vi "Helmholtz2D_FEM_Check Input_RHS.vi"(8 "error in (no error)":errorcluster, 10 "Grid":cluster{"Xi":dbl[], "Yi":dbl[]}, 11 "F(x, y)":dbl[](array[numeric])) -> (0 "error out":errorcluster)   [LabVIEW 2017, in "NI_PDE.lvlib"]
uses:
  <vilib>/gmath/NI_PDE.lvlib
  <vilib>/gmath/pde.llb/Common/PDE_Error.ctl
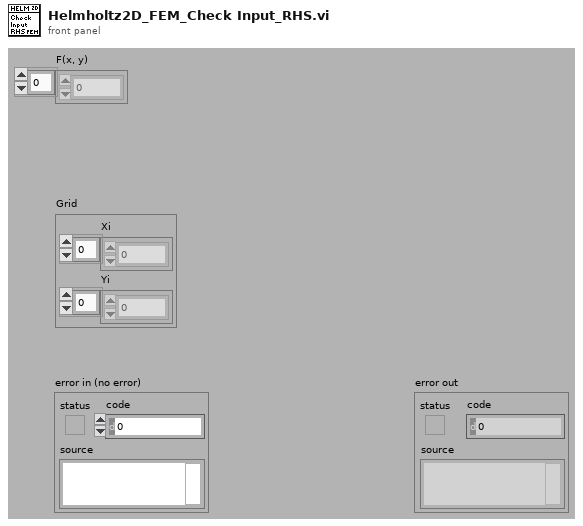
[diagram p1: front panel]
types:
  T1 = typedef "NI_PDE.lvlib/PDE_Error.ctl" = enum16{"No Error", "k is zero", "End point <= start point", "# of time steps < 2", "# of spatial points < 3", "# of grid < 1 for FEM", "# of boundary < 3 for FEM", "Incompatible RHS size", "Incompatible BC size", "Incompatible IC size", "PDE class conflict", "RHS class conflict", "Domain class conflict", "BC class conflict", "IC class conflict"}
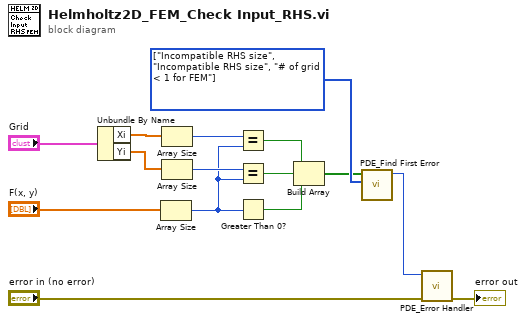
[diagram p0: block diagram]
diagram:
  w11 = T1[] [enum."Incompatible RHS size", enum."Incompatible RHS size", enum."# of grid < 1 for FEM"] items=["No Error", "k is zero", "End point <= start point", "# of time steps < 2", "# of spatial points < 3", "# of grid < 1 for FEM", "# of boundary < 3 for FEM", "Incompatible RHS size", "Incompatible BC size", "Incompatible IC size", "PDE class conflict", "RHS class conflict", "Domain class conflict", "BC class conflict", "IC class conflict"]
  n1 = Unbundle By Name("Grid") -> ("Xi"=w9:dbl[], "Yi"=w8:dbl[])
  n2 = Array Size(array="F(x, y)") -> (size(s)=w1:i32)
  n3 = Array Size(array=w9) -> (size(s)=w6:i32)
  n4 = Array Size(array=w8) -> (size(s)=w7:i32)
  n5 = Equal?(x=w6, y=w1) -> (x = y?=w5:bool)
  n6 = Equal?(x=w7, y=w1) -> (x = y?=w4:bool)
  n7 = Greater Than 0?(x=w1) -> (x > 0?=w3:bool)
  n8 = Build Array(w5, w4, w3) -> (w2:bool[])
  n9 = call <vilib>:"PDE_Find First Error.vi"("PDE Error"=w11, "Failure"=w2) -> ("first error"=w12:T1)  [unwired: 9 out]
  n10 = call <vilib>:"PDE_Error Handler.vi"("error in (no error)"="error in (no error)", "PDE error"=w12) -> ("error out"=→"error out":errorcluster)  [unwired: 9 out]
